vi "Test Clock.vi"(9 "Set Time":i32, 11 "Command":T1) -> (1 "Running?":bool, 3 "Time":i32)   [LabVIEW 2015]
uses:
  Clock Control Enum.ctl
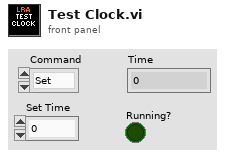
[diagram p1: front panel]
types:
  T1 = typedef "Clock Control Enum.ctl" = enum16{"Set", "Get", "Start", "Stop"}
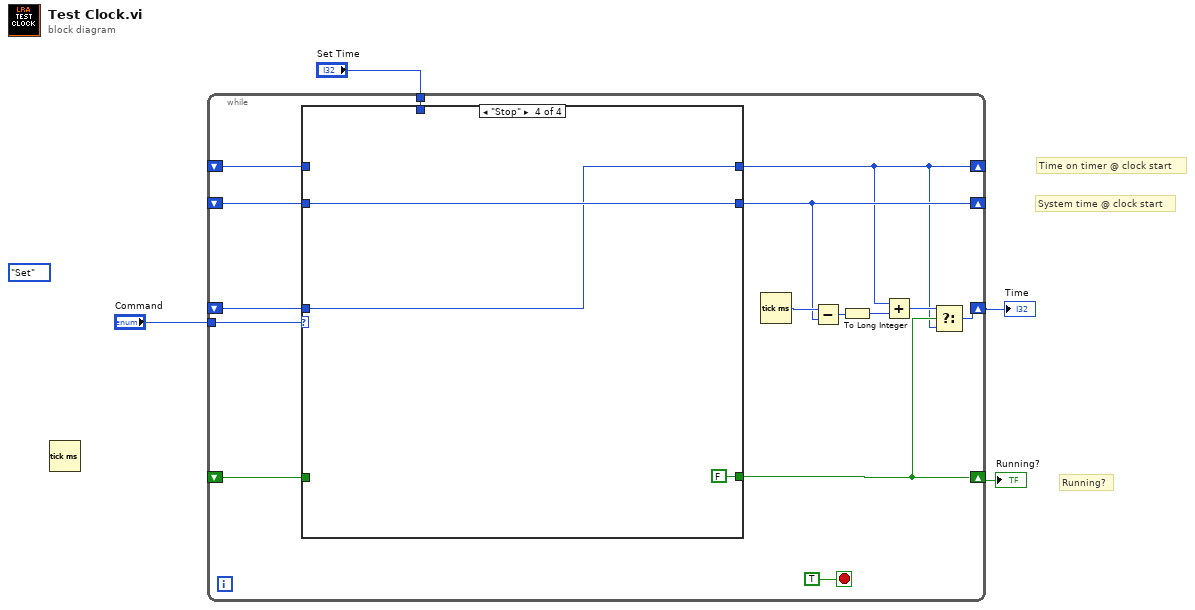
[diagram p0: block diagram]
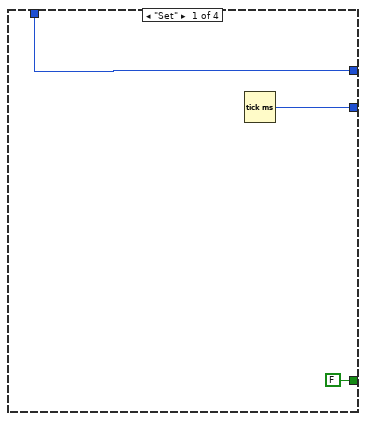
[diagram p2: hidden frame]
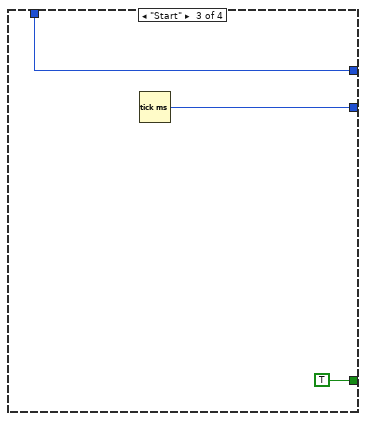
[diagram p4: hidden frame]
diagram:
  (unwired) Clock_Control_Enum."Set"
  # "Running?"
  # "Time on timer @ clock start"
  # "System time @ clock start"
  n1 = Tick Count (ms)() -> ()  [unwired: 1 out]
  n2 = while {
    shift-right: [w12] -> _
    shift-left: _ -> [w18]
    tunnel: "Command" -> [w17]
    shift-right: [w6] -> _
    shift-left: _ -> [w16]
    shift-right: [w9] -> w2
    shift-left: _ -> [w11]
    tunnel: "Set Time" -> [w10]
    shift-right: [w7] -> w3
    shift-left: _ -> [w5]
    stop <- TRUE stop-if-true
    n3 = case shown="\"Stop\"" w17 {
      tunnel: [w22 w24 w28 w30] -> w12
      tunnel: w18 -> [_ w24 _ w30]
      tunnel: [w20 w25 w26 w29] -> w6
      tunnel: w16 -> [_ w25 _ _]
      tunnel: w11 -> [_ w23 _ _]
      tunnel: [FALSE w23 TRUE FALSE] -> w9
      tunnel: w10 -> [w20 _ w26 _]
      tunnel: w5 -> [_ _ _ w29]
      frame "Set" {
        n4 = Tick Count (ms)() -> (millisecond timer value=w22:u32)
      }
      frame "Get", Default {
      }
      frame "Start" {
        n5 = Tick Count (ms)() -> (millisecond timer value=w28:u32)
      }
      frame "Stop" {
      }
    }
    n6 = Tick Count (ms)() -> (millisecond timer value=w15:u32)
    n7 = Subtract(x=w15, y=w12) -> (x-y=w14:u32)
    n8 = To Long Integer(number=w14) -> (32bit integer=w13:i32)
    n9 = Add(x=w6, y=w13) -> (x+y=w8:i32)
    n10 = Select(t=w8, s=w9, f=w6) -> (s? t:f=w7:i32)
  }
  "Time" <- w3
  "Running?" <- w2
